vi "Calculation lg.vi"(9 "Save path":path=path "J:/20160720 陈老师 谷粒 米粒实验/binary&分割图/提取数据/谷粒米粒综合 +计算平均反射率.txt", 11 "file path (dialog if empty)":path=path "J:/20160720 陈老师 谷粒 米粒实验/binary&分割图/提取数据/谷粒米粒综合 +计算平均反射率.txt") -> ()   [LabVIEW 2015]
uses:
  <vilib>/Utility/file.llb/Read Delimited Spreadsheet (string).vi
  <vilib>/Utility/file.llb/Write Delimited Spreadsheet (string).vi
panel:
  out "output array 2":string[][](array[string])
  out "all rows":string[][](array[string])
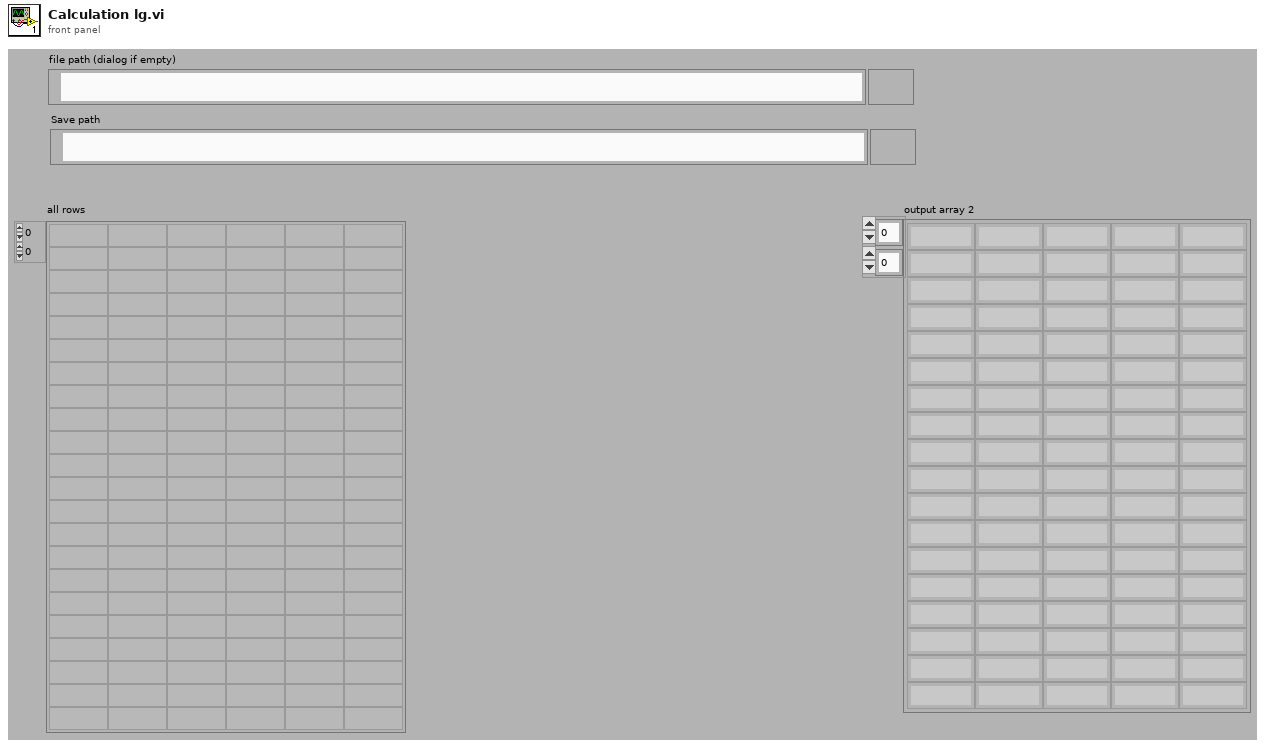
[diagram p1: front panel]
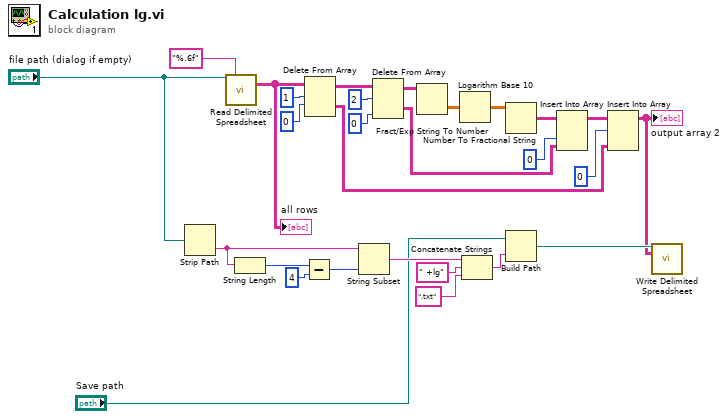
[diagram p0: block diagram]
diagram:
  n1 = Strip Path(path="file path (dialog if empty)") -> (name=w23:string)  [unwired: 1 out]
  n2 = call-poly <vilib>:"Read Delimited Spreadsheet.vi"("file path (dialog if empty)"="file path (dialog if empty)", "format (%s)"="%.6f" ("format (%.3f)")) -> ("all rows"=w3:string[][])  [unwired: 8 in, 5 out]
  "all rows" <- w3
  n3 = String Length(string=w23) -> (length=w22:i32)
  n4 = Subtract(x=w22, y=4) -> (x-y=w20:i32)
  n5 = Delete From Array(array=w3, length=1, index (row)=0) -> (deleted portion=w12:string[][], array with subset deleted=w25:string[][])  [unwired: 1 in]
  n6 = String Subset(string=w23, length (rest)=w20) -> (substring=w9:string)  [unwired: 1 out]
  n7 = Delete From Array(array=w25, length=2, index (col)=0 ("index")) -> (deleted portion=w7:string[][], array with subset deleted=w4:string[][])  [unwired: 1 in]
  n8 = Fract/Exp String To Number(string=w4) -> (number=w6:dbl[][])  [unwired: 4 out]
  n9 = Logarithm Base 10(1:w6) -> (0:w5:dbl[][])
  n10 = Concatenate Strings(w9, " +lg" ("string"), ".txt" ("string")) -> (w19:string)
  n11 = Number To Fractional String(number=w5) -> (F-format string=w14:string[][])  [unwired: 3 out]
  n12 = Build Path(base path="Save path", name or relative path=w19) -> (appended path=w17:path)
  n13 = Insert Into Array(array=w14, index (col)=0 ("index"), new element=w7) -> (w13:string[][])  [unwired: 1 in]
  n14 = Insert Into Array(array=w13, index (row)=0, new element=w12) -> (w2:string[][])  [unwired: 1 in]
  "output array 2" <- w2
  n15 = call-poly <vilib>:"Write Delimited Spreadsheet.vi"("file path (dialog if empty)"=w17, "2D data"=w2) -> ()  [unwired: 12 in, 2 out]
